vi "YAML_int.vi"(1 "value":i64, 2 "name":string) -> (0 "result":string)   [LabVIEW 2011]
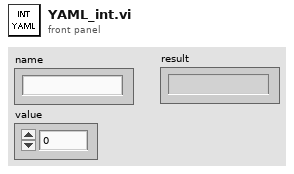
[diagram p1: front panel]
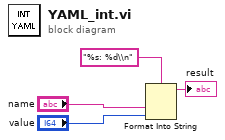
[diagram p0: block diagram]
diagram:
  n1 = Format Into String(format string="%s: %d\\n", "name", "value") -> (resulting string=→"result":string)  [unwired: 2 in, 1 out]
